vi "Command Drive Distance Field (Gyro Hold, Sensor Stop).vi"(2 "Input Robot System Funtions":T1, 3 "Cmd Parameter 1":dbl, 4 "Cmd Parameter 2":dbl, 5 "Startup":bool) -> (0 "Output Robot System Functions":T1, 1 "Completed":bool)   [LabVIEW 2014]
uses:
  Subsystems VIs/Robot Commands.ctl
  Command Execution State.ctl
  Global Variables/Sensor Data (Edited).vi
  Global Variables/Settings.vi
panel:
  out "PID Tracking":cluster{"Goal Wheel Position":dbl, dbl}(graph)={"Goal Wheel Position"=0.0, -90.17571233858979}
  # "Sample robot\ncontrol output.\nReplace with \nactual teleop \ncontrol signal \nstructure."
  # "Field Centric"
  # "Field Centric"
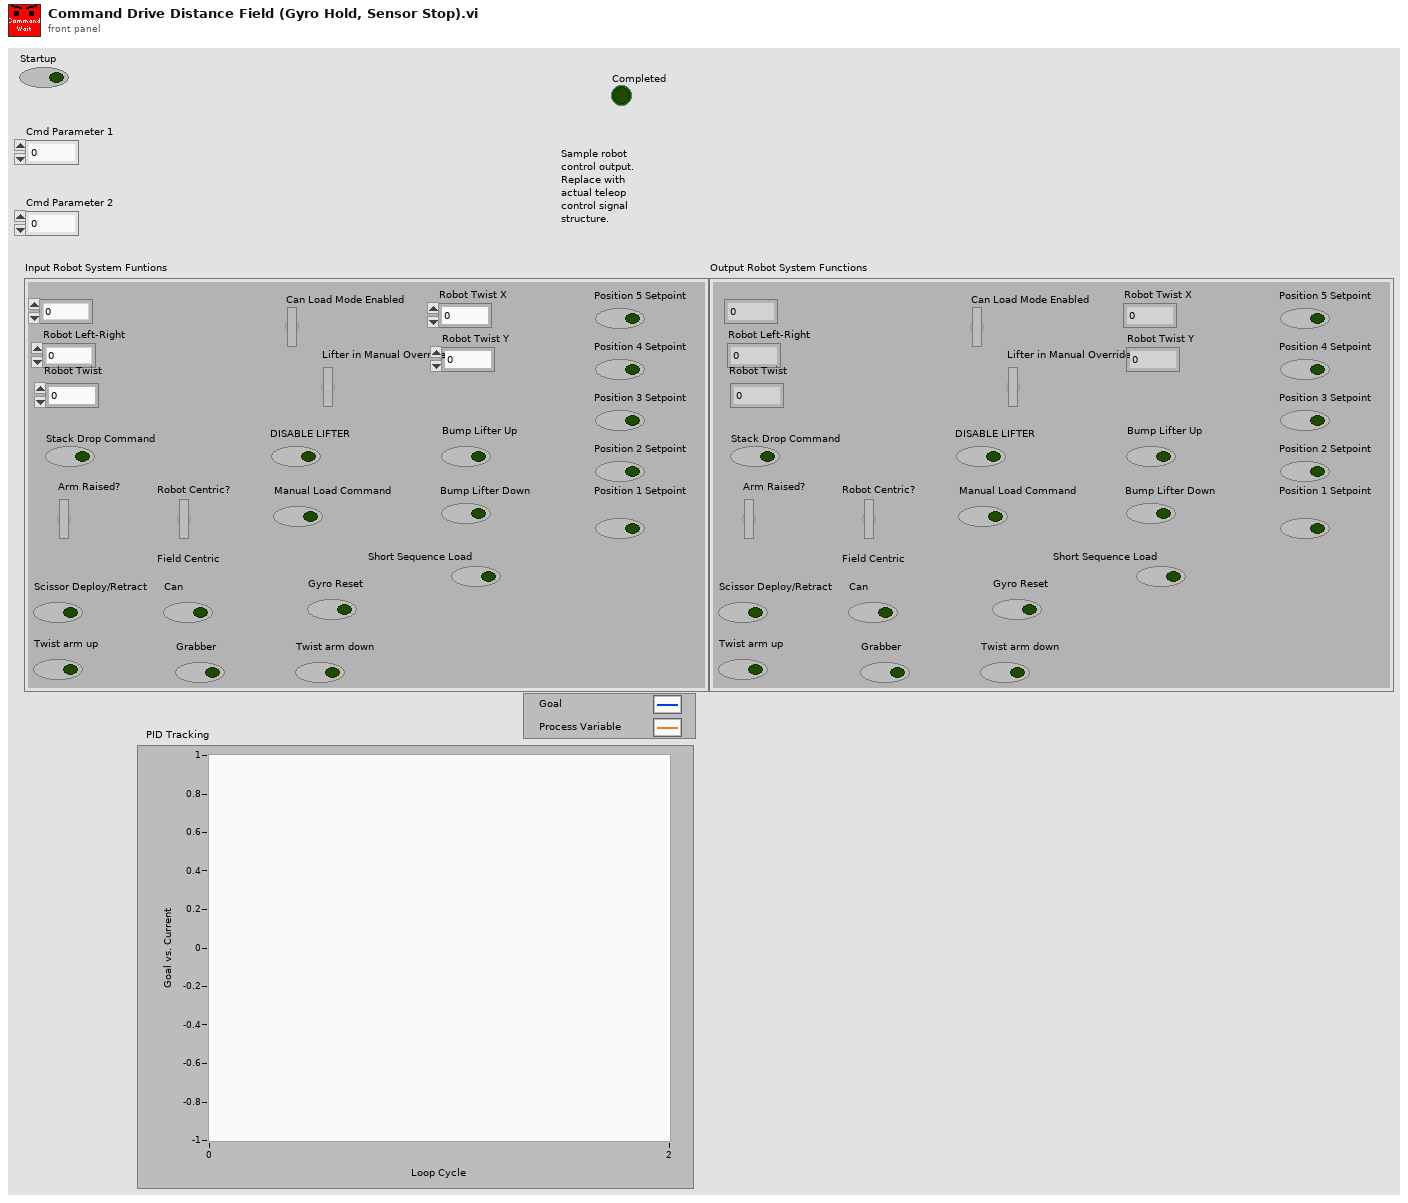
[diagram p1: front panel]
types:
  T1 = typedef "Robot Commands.ctl" = cluster{"Robot Forward-Reverse":dbl, "Robot Left-Right":dbl, "Robot Twist":dbl, "Can Load Mode Enabled":bool, "Lifter in Manual Override?":bool, "Stack Drop Command":bool, "Arm Raised?":bool, "DISABLE LIFTER":bool, "Position 1 Setpoint":bool, "Position 2 Setpoint":bool, "Position 3 Setpoint":bool, "Position 4 Setpoint":bool, "Position 5 Setpoint":bool, "Bump Lifter Down":bool, "Bump Lifter Up":bool, "Manual Load Command":bool, "Robot Centric?":bool, "Scissor Deploy/Retract":bool, "Grabber":bool, "Can":bool, "Twist arm up":bool, "Gyro Reset":bool, "Twist arm down":bool, "Short Sequence Load":bool, "Robot Twist X":dbl, "Robot Twist Y":dbl}
  T2 = typedef "Command Execution State.ctl" = enum16{"Initialize", "Execute", "Finish"}
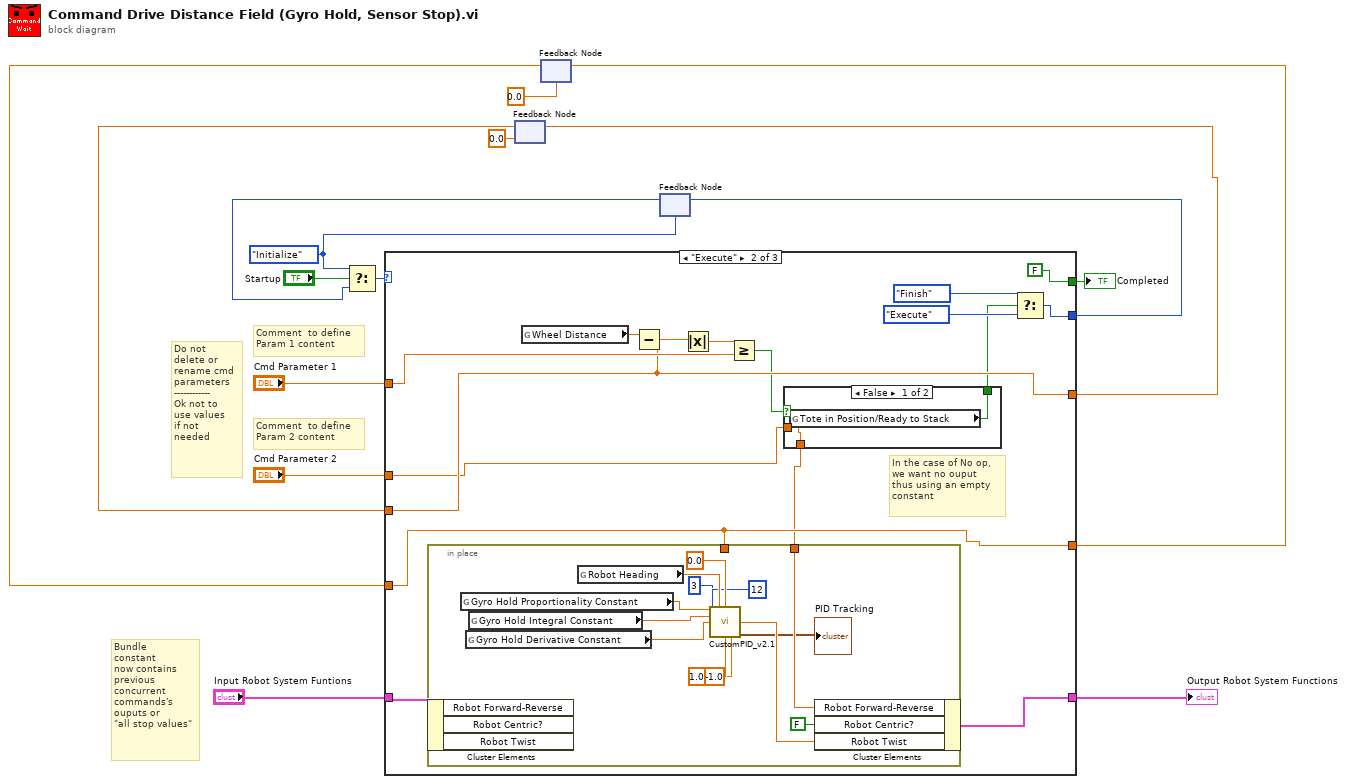
[diagram p0: block diagram]
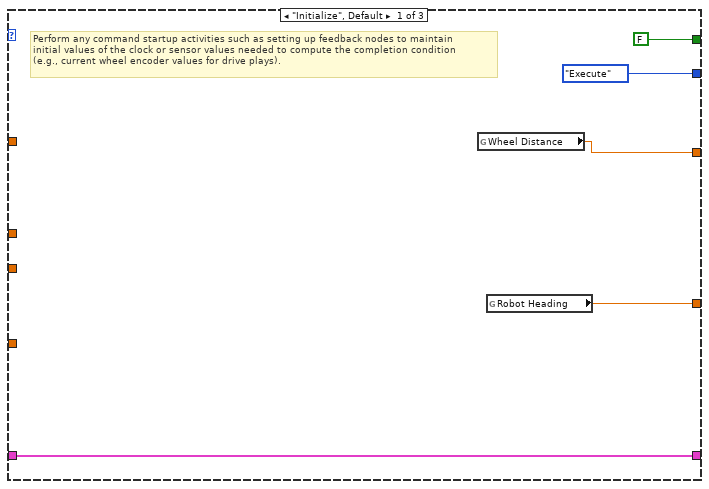
[diagram p2: hidden frame]
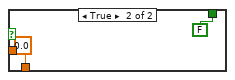
[diagram p3: hidden frame]
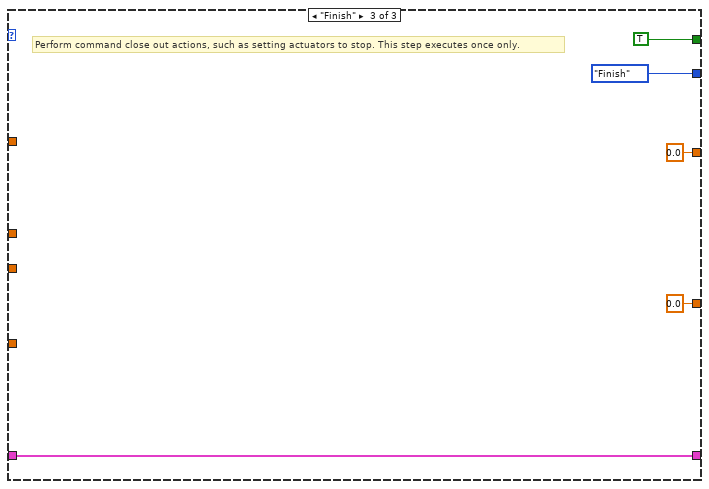
[diagram p4: hidden frame]
diagram:
  w11 = Command_Execution_State."Initialize" ("Play State")
  # "Bundle \nconstant\nnow contains\nprevious \nconcurrent\ncommands's\nouputs or\n\"all stop values\""
  # "Do not \ndelete or\nrename cmd\nparameters\n------------\nOk not to \nuse values\nif not \nneeded"
  # "Comment  to define\nParam 2 content"
  # "Comment  to define\nParam 1 content"
  n1 = feedback #1(0.0 ("Wheel Distance")) -> (w5:dbl)
  n2 = feedback #2(0.0 ("Wheel Distance")) -> (w2:dbl)
  n3 = feedback #3(w11) -> (w12:T2)
  n4 = Select(t=w11, s="Startup", f=w12) -> (s? t:f=w16:T2)
  n5 = case shown="\"Execute\"" w16 {
    tunnel: [FALSE FALSE TRUE] -> w14
    tunnel: [Command_Execution_State."Execute" ("Play State") w28 Command_Execution_State."Finish" ("f")] -> w13
    tunnel: "Cmd Parameter 1" -> [_ w30 _]
    tunnel: "Cmd Parameter 2" -> [_ w23 _]
    tunnel: [w19 w31 w55] -> w7
    tunnel: "Input Robot System Funtions" -> [w19 w32 w55]
    tunnel: [w18 w29 0.0 ("Wheel Distance")] -> w6
    tunnel: w5 -> [_ w29 _]
    tunnel: [w17 w26 0.0 ("Wheel Distance")] -> w3
    tunnel: w2 -> [_ w26 _]
    frame "Initialize", Default {
      # "Perform any command startup activities such as setting up feedback nodes to maintain \ninitial values of the clock or sensor values needed to compute the completion condition\n(e.g., current wheel encoder values for drive plays)."
      n6 = global read "Sensor Data (Edited).vi" "Wheel Distance"() -> (w18:dbl)
      n7 = global read "Sensor Data (Edited).vi" "Robot Heading"() -> (w17:dbl)
    }
    frame "Execute" {
      # "In the case of No op, \nwe want no ouput \nthus using an empty \nconstant"
      n8 = global read "Sensor Data (Edited).vi" "Wheel Distance"() -> (w37:dbl)
      n9 = Subtract(x=w37, y=w29) -> (x-y=w34:dbl)
      n10 = Absolute Value(x=w34) -> (abs(x)=w33:dbl)
      n11 = Greater Or Equal?(x=w33, y=w30) -> (x >= y?=w25:bool)
      n12 = case shown="False" w25 {
        tunnel: [w39 FALSE ("Tote in Position/Ready to Stack")] -> w24
        tunnel: w23 -> [w38 _]
        tunnel: [w38 0.0 ("Cmd Parameter 2")] -> w22
        frame False {
          n13 = global read "Sensor Data (Edited).vi" "Tote in Position/Ready to Stack"() -> (w39:bool)
        }
        frame True {
        }
      }
      n14 = in-place {
        in-place-border: w22 -> [w54]
        in-place-border: w26 -> [_]
        n15 = in-place-cluster #4(w32) -> ()  [unwired: 3 out]
        n16 = global read "Settings.vi" "Gyro Hold Proportionality Constant"() -> (w45:dbl)
        n17 = global read "Settings.vi" "Gyro Hold Derivative Constant"() -> (w43:dbl)
        n18 = global read "Settings.vi" "Gyro Hold Integral Constant"() -> (w44:dbl)
        n19 = global read "Sensor Data (Edited).vi" "Robot Heading"() -> (w51:dbl)
        n20 = call "CustomPID_v2.1.vi"("Kp"=w45, "Process Variable"=w51, "Goal"=0.0 ("Setpoint"), "Ki"=w44, "Kd"=w43, "N-Diff"=3, "N-Int"=12, "Max Ouput"=1.0, "Min Output"=-1.0) -> ("Command"=w52:dbl, "PID Tracking"=→"PID Tracking":cluster{"Goal Wheel Position":dbl, dbl})  [unwired: 4 in, 1 out]
        n21 = in-place-cluster #4("Robot Forward-Reverse"=w54, "Robot Centric?"=FALSE, "Robot Twist"=w52) -> (w31:T1)
      }
      n22 = Select(t=Command_Execution_State."Finish" ("Play State"), s=w24, f=Command_Execution_State."Execute" ("Play State")) -> (s? t:f=w28:T2)
    }
    frame "Finish" {
      # "Perform command close out actions, such as setting actuators to stop. This step executes once only."
    }
  }
  "Completed" <- w14
  "Output Robot System Functions" <- w7
  n23 = feedback-in #1(w6) -> ()
  n24 = feedback-in #2(w3) -> ()
  n25 = feedback-in #3(w13) -> ()
